vi "ReadI2C.vi"(8 "error in (no error)":errorcluster, 9 "Num Bytes to Fetch (64)":u16=64 min=1, 10 "Slave Address (0x57)":u16=87 format="%.0x") -> (0 "error out":errorcluster, 2 "Incoming Data":u8[](array[numeric]) format="%.0x")   [LabVIEW 2024]
panel:
  out "Aardvark Handle 1":i32
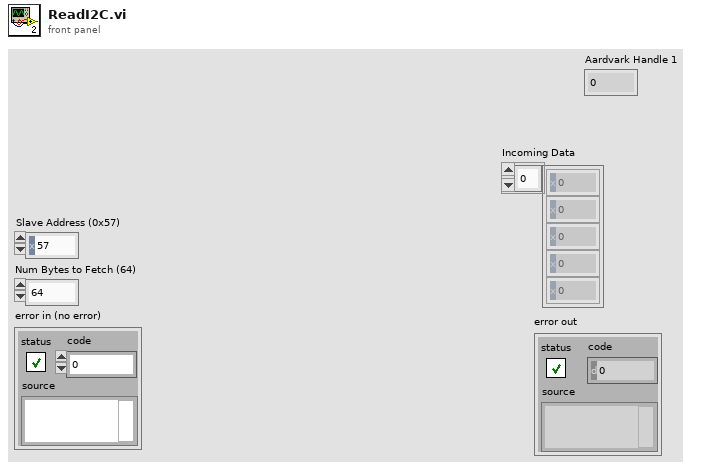
[diagram p1: front panel]
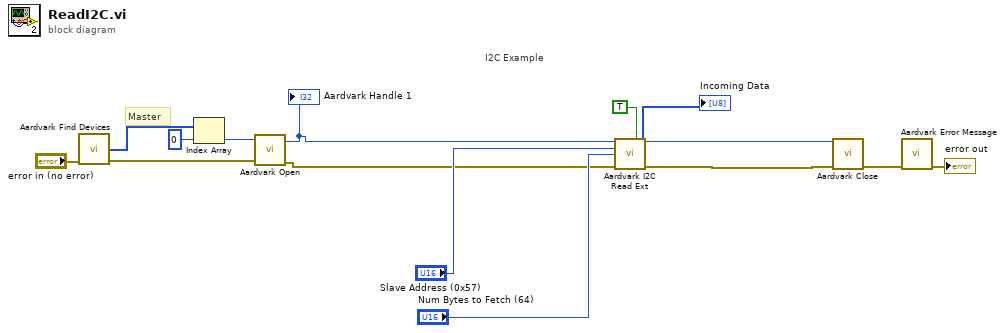
[diagram p0: block diagram]
diagram:
  # "Master"
  # "I2C Example"
  n1 = call <instrlib>:"Aardvark Find Devices.vi"("error in (no error)"="error in (no error)") -> ("Ports"=w8:u16[], "error out"=w12:errorcluster)  [unwired: 12 in, 1 out]
  n2 = Index Array(array=w8, index=0) -> (element=w14:u16)
  n3 = call <instrlib>:"Aardvark Open.vi"("Port Number (0)"=w14, "error in (no error)"=w12) -> ("Aardvark Handle"=w7:i32, "error out"=w4:errorcluster)  [unwired: 12 in]
  "Aardvark Handle 1" <- w7
  n4 = call <instrlib>:"Aardvark I2C Read Ext.vi"("Aardvark Handle"=w7, "No Stop? (False)"=TRUE, "Address (0x50)"="Slave Address (0x57)", "Num Bytes to Fetch (64)"="Num Bytes to Fetch (64)", "error in (no error)"=w4) -> ("dup Aardvark Handle"=w9:i32, "Incoming Data"=→"Incoming Data":u8[], "error out"=w3:errorcluster)  [unwired: 7 in, 1 out]
  n5 = call <instrlib>:"Aardvark Close.vi"("Aardvark Handle"=w9, "error in (no error)"=w3) -> ("error out"=w13:errorcluster)  [unwired: 13 in]
  n6 = call <instrlib>:"Aardvark Error Message.vi"("error in (no error)"=w13) -> ("error out"=→"error out":errorcluster)  [unwired: 10 in, 4 out]
